vi "Get Lockin Parameters.vi"(8 "error in (no error)":errorcluster, 11 "RP Instrument in":refnum<class "RP Instrument.lvclass">) -> (0 "error out":errorcluster, 2 "Lockin parameters":T1={"Frequency"=0.0, "Phase"=0.0, "Syncronous"=FALSE, "Points per sine wave"=0, "DDS"=FALSE, "Frequency word"=0, "Phase word"=0, "DDS modulus"=15120, "DDS clock"=125000000.0} {"DDS clock" format="%_17pHz"; "DDS modulus" format="0x%x (%d)"; "Phase" format="%#_gdeg"; "Frequency" format="%_17pHz"}, 3 "RP Instrument out":refnum<class "RP Instrument.lvclass">)   [LabVIEW 2024]
uses:
  RP Instrument.lvclass
  SoftwareLockin/Lockin Parameters.ctl
  RP Status Offsets.ctl
  RP Instrument.lvclass/RP Instrument.ctl
  RP Communicator/RP Communicator.lvclass
panel:
  out "Phase out 1":u32=1 format="0x%x (%d)"
  out "Phase out 2":u32=1 format="0x%x (%d)"
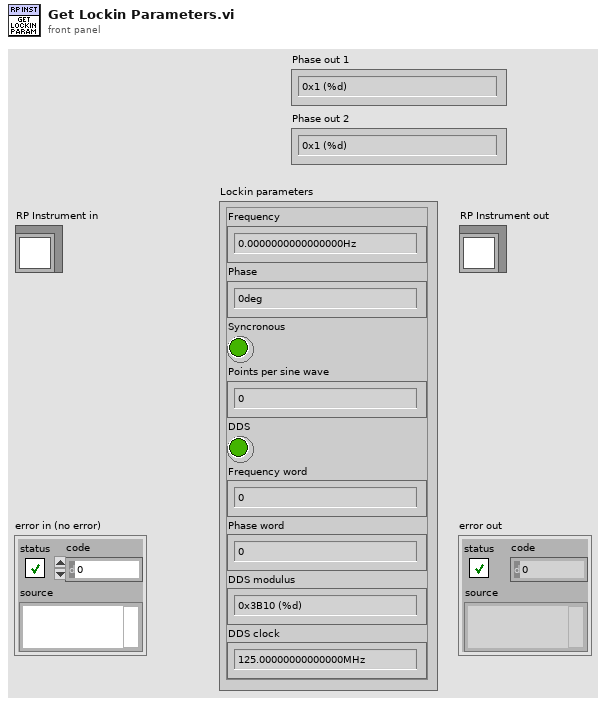
[diagram p1: front panel]
types:
  T1 = typedef "Lockin Parameters.ctl" = cluster{"Frequency":dbl, "Phase":dbl, "Syncronous":bool, "Points per sine wave":i32, "DDS":bool, "Frequency word":u32, "Phase word":u32, "DDS modulus":i64, "DDS clock":dbl}
  T2 = typedef "RP Status Offsets.ctl" = u16
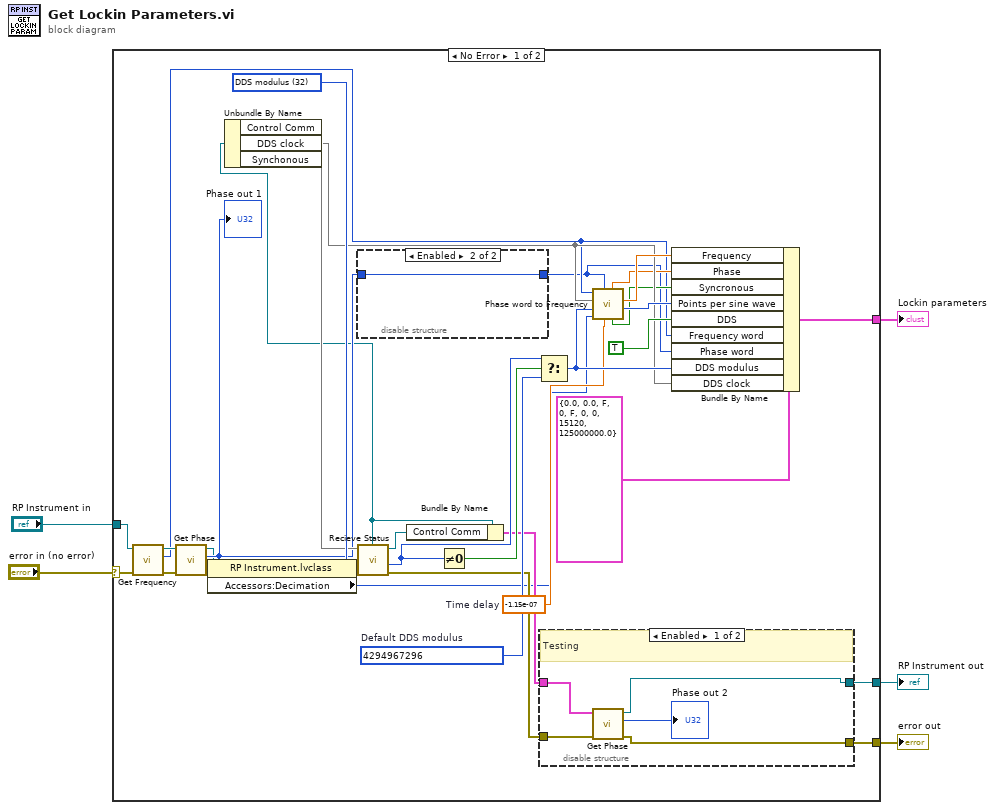
[diagram p0: block diagram]
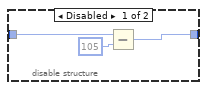
[diagram p3: hidden frame]
diagram:
  n1 = case shown="No Error" "error in (no error)" {
    selector: "error in (no error)" -> [w21 w50]
    tunnel: [w13 w50] -> w4
    tunnel: [w11 w49] -> w2
    tunnel: "RP Instrument in" -> [w15 w49]
    tunnel: [w27 _] -> w1
    frame No Error {
      w16 = -1.15e-07  # Time delay
      w33 = i64 4294967296  # Default DDS modulus
      w37 = T2 32 items=["Writer address"=0, "Record start position"=4, "Trig state and ID"=8, "Phase"=12, "X1"=16, "Y1"=20, "RxFIFO counter or  X2"=24, "TxFIFO counter or Y2"=28, "DDS modulus"=32] ("Status offsets")
      n2 = call-dynamic "Get Frequency.vi"("error in (no error)"=w21, "RP Instrument in"=w15) -> ("error out"=w32:errorcluster, "Frequency"=w18:u32, "RP Instrument out"=w31:refnum<class "RP Instrument.lvclass">)  [unwired: 7 in]
      n3 = call-dynamic "Get Phase.vi"("error in (no error)"=w32, "RP Instrument in"=w31) -> ("error out"=w30:errorcluster, "Phase"=w10:u32, "RP Instrument out"=w8:refnum<class "RP Instrument.lvclass">)  [unwired: 7 in]
      "Phase out 1" <- w10
      n4 = property class="RP Instrument.lvclass"(reference=w8, error in=w30) -> (reference out=w7:refnum<class "RP Instrument.lvclass">, error out=w9:errorcluster, "Accessors:Decimation"=w6:i32)
      n5 = Unbundle By Name(w7) -> ("Control Comm"=w36, "DDS clock"=w23)  [unwired: 1 out]
      n6 = disable-structure shown="Enabled" {
        disable-tunnel: w10 -> [w47 w48]
        disable-tunnel: [w46 w48] -> w17
        frame Disabled {
          n7 = Subtract(x=w47, y=u32 105) -> (x-y=w46:u32)
        }
        frame Enabled {
        }
      }
      n8 = call-dynamic "Recieve Status.vi"("error in (no error)"=w9, "Status offset"=w37, "RP Communicator in"=w36) -> ("error out"=w14:errorcluster, "Status response"=w34:u32, "RP Communicator out"=w22:refnum<class "RP Communicator.lvclass">)  [unwired: 6 in]
      n9 = Bundle By Name(cluster=w7, "Control Comm"=w22) -> (w12:cluster{})
      n10 = Not Equal To 0?(x=w34) -> (x != 0?=w35:bool)
      n11 = Select(t=w34, s=w35, f=w33) -> (s? t:f=w24:i64)
      n12 = disable-structure shown="Enabled" {
        disable-tunnel: w14 -> [w42 w43]
        disable-tunnel: [w41 w43] -> w13
        disable-tunnel: w12 -> [w40 w44]
        disable-tunnel: [w39 w44] -> w11
        frame Enabled {
          # "Testing"
          n13 = call-dynamic "Get Phase.vi"("error in (no error)"=w42, "RP Instrument in"=w40) -> ("error out"=w41:errorcluster, "Phase"=→"Phase out 2":u32, "RP Instrument out"=w39:refnum<class "RP Instrument.lvclass">)  [unwired: 7 in]
        }
        frame Disabled {
        }
      }
      n14 = call "Phase word to Frequency.vi"("Time delay"=w16, "Phase word"=w17, "Decimation"=w6, "DDS modulus"=w24, "DDS clock"=w23, "Frequency word"=w18) -> ("Points per sine wave"=w26:u64, "Actual frequency"=w28:dbl, "Syncronous"=w20:bool, "Phase"=w19:dbl)  [unwired: 2 in]
      n15 = Bundle By Name(cluster=T1 {"Frequency"=0.0, "Phase"=0.0, "Syncronous"=FALSE, "Points per sine wave"=0, "DDS"=FALSE, "Frequency word"=0, "Phase word"=0, "DDS modulus"=15120, "DDS clock"=125000000.0} ("Lockin parameters"), "Frequency"=w28, "Phase"=w19, "Syncronous"=w20, "Points per sine wave"=w26, "DDS"=TRUE, "Frequency word"=w18, "Phase word"=w17, "DDS modulus"=w24, "DDS clock"=w23) -> (w27:T1)
    }
    frame Error {
    }
  }
  "error out" <- w4
  "RP Instrument out" <- w2
  "Lockin parameters" <- w1
